vi "bk 9130 Error Query.vi"(8 "error in (no error)":errorcluster, 11 "VISA resource name":refnum<visa-resource-name>) -> (0 "error out":errorcluster, 1 "Error Message":string, 2 "Error Code":i32[](array[numeric]), 3 "VISA resource name out":refnum<visa-resource-name>)   [LabVIEW 2009]
doc: "This VI queries the instrument for any errors in the instrument's error queue. It will continue to read errors until all errors have been read from the instrument. Any errors will be returned in the Error Out cluster.\n\nNote:\nThis VI is called automatically by most driver VIs so it is not usually necessary to call this in an application."
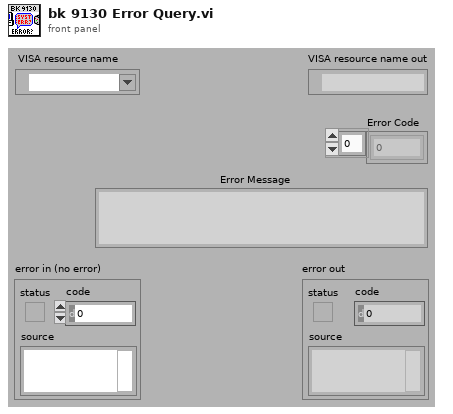
[diagram p1: front panel]
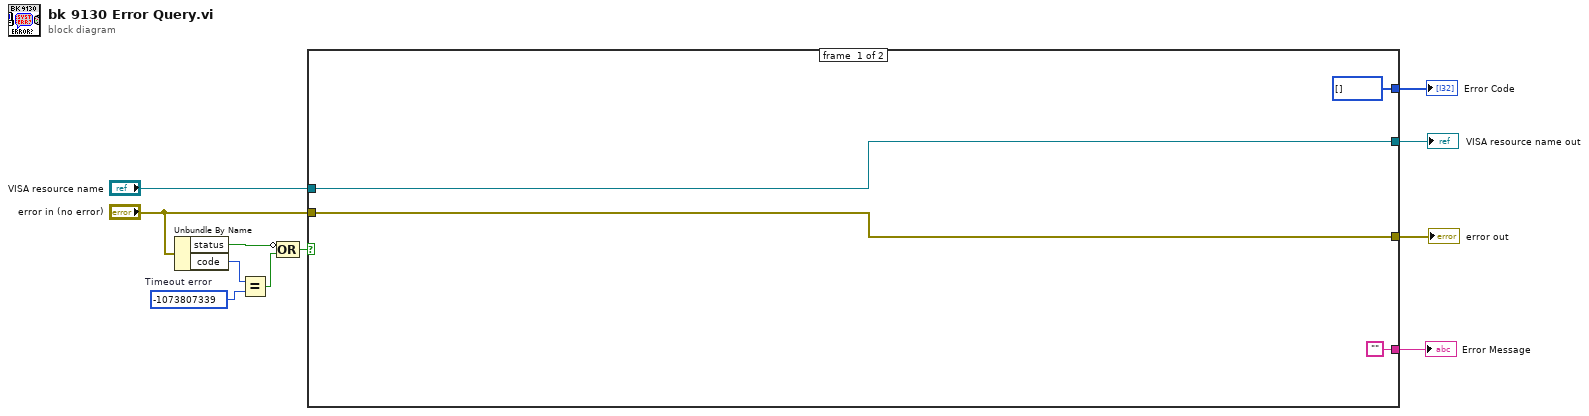
[diagram p0: block diagram]
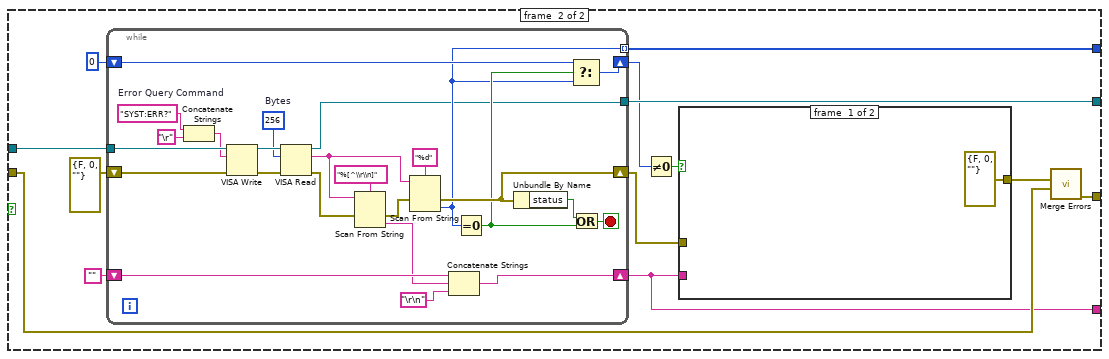
[diagram p2: hidden frame]
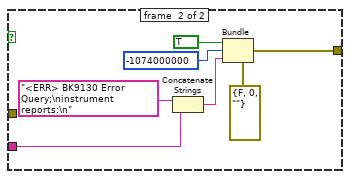
[diagram p3: hidden frame]
diagram:
  w8 = -1073807339  # Timeout error
  n1 = Unbundle By Name("error in (no error)") -> ("status"=w9:bool, "code"=w6:i32)
  n2 = Equal?(x=w6, y=w8) -> (x = y?=w7:bool)
  n3 = Compound Arithmetic op=OR(invert w9, w7) -> (w5:bool)
  n4 = case shown="True" w5 {
    tunnel: [w15 w28] -> w2
    tunnel: "VISA resource name" -> [w15 w27]
    tunnel: "error in (no error)" -> [w14 w21]
    tunnel: [w14 w25] -> w1
    tunnel: ["" w18] -> w4
    tunnel: [i32[] [] w17] -> w3
    frame #0 {
    }
    frame #1 {
      n5 = while {
        tunnel: [w38] -> w17 mode=indexing
        shift-left: errorcluster {"status"=FALSE, "code"=0, "source"=""} ("error in (no error)") -> [w43]
        shift-right: [w42] -> w16
        shift-left: 0 -> [w45]
        shift-right: [w44] -> w19
        shift-left: "" -> [w49]
        shift-right: [w46] -> w18
        tunnel: w27 -> [w53]
        tunnel: [w35] -> w28
        stop <- w51 stop-if-true
        w34 = u32 256  # Bytes
        w31 = "SYST:ERR?"  # Error Query Command
        n6 = Concatenate Strings(w31, "\r") -> (w30:string)
        n7 = VISA Write(VISA resource name=w53, write buffer=w30, error in (no error)=w43) -> (VISA resource name out=w37:refnum<visa-resource-name>, error out=w36:errorcluster)  [unwired: 1 out]
        n8 = VISA Read(VISA resource name=w37, byte count=w34, error in (no error)=w36) -> (VISA resource name out=w35:refnum<visa-resource-name>, read buffer=w32:string, error out=w33:errorcluster)  [unwired: 1 out]
        n9 = Scan From String(format string="%[^\\r\\n]", input string=w32, error in=w33) -> (error out=w41:errorcluster, output 1=w47:string)  [unwired: 2 in, 2 out]
        n10 = Scan From String(format string="%d", input string=w32, error in=w41) -> (error out=w42:errorcluster, output 1=w38:i32)  [unwired: 2 in, 2 out]
        n11 = Concatenate Strings(w49, w47, "\r\n") -> (w46:string)
        n12 = Equal To 0?(x=w38) -> (x = 0?=w39:bool)
        n13 = Unbundle By Name(w42) -> ("status"=w40:bool)
        n14 = Select(t=w45, s=w39, f=w38) -> (s? t:f=w44:i32)
        n15 = Or(x=w40, y=w39) -> (x .or. y?=w51:bool)
      }
      n16 = Not Equal To 0?(x=w19) -> (x != 0?=w23:bool)
      n17 = case shown="False" w23 {
        tunnel: w18 -> [_ w57]
        tunnel: [errorcluster {"status"=FALSE, "code"=0, "source"=""} ("error out") w56] -> w22
        tunnel: w16 -> [_ _]
        frame #0 {
        }
        frame #1 {
          n18 = Concatenate Strings("<ERR> BK9130 Error Query;\ninstrument reports:\n" ("Source"), w57) -> (w58:string)
          n19 = Bundle(cluster=errorcluster {"status"=FALSE, "code"=0, "source"=""} ("error out"), "status"=TRUE ("Status"), "code"=-1074000000 ("Code"), "source"=w58) -> (w56:errorcluster)
        }
      }
      n20 = call <vilib>:"Merge Errors.vi"("error in 3 (no error)"=w21, "error in 2 (no error)"=w22) -> ("error out"=w25:errorcluster)  [unwired: 5 in]
    }
  }
  "VISA resource name out" <- w2
  "error out" <- w1
  "Error Message" <- w4
  "Error Code" <- w3
